vi "Drive Train Charts.vi"() -> ()   [LabVIEW 2016]
uses:
  <vilib>/Rock Robotics/Network Tables/NT Read Number.vi
panel:
  out "Right Target":dbl(graph)
  out "Right Throttle":dbl(graph)
  out "Right Velocity":dbl(graph)
  out "Right Current":dbl(graph)
  out "Left Target":dbl(graph)
  out "Left Throttle":dbl(graph)
  out "Left Velocity":dbl(graph)
  out "Left Current":dbl(graph)
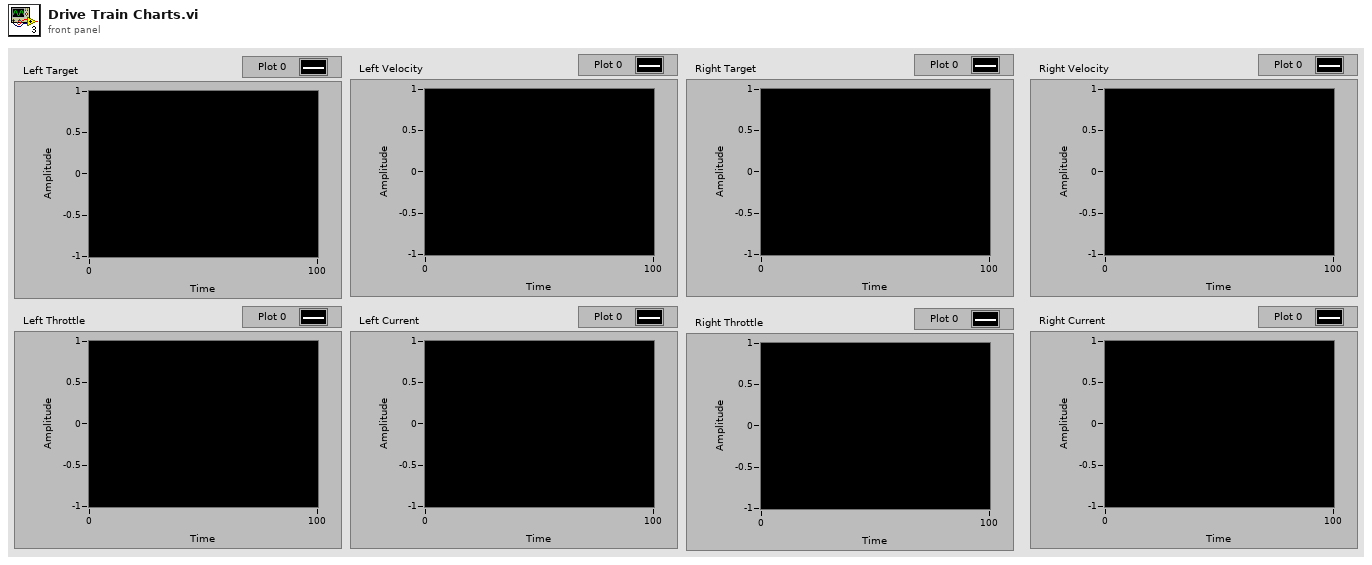
[diagram p1: front panel]
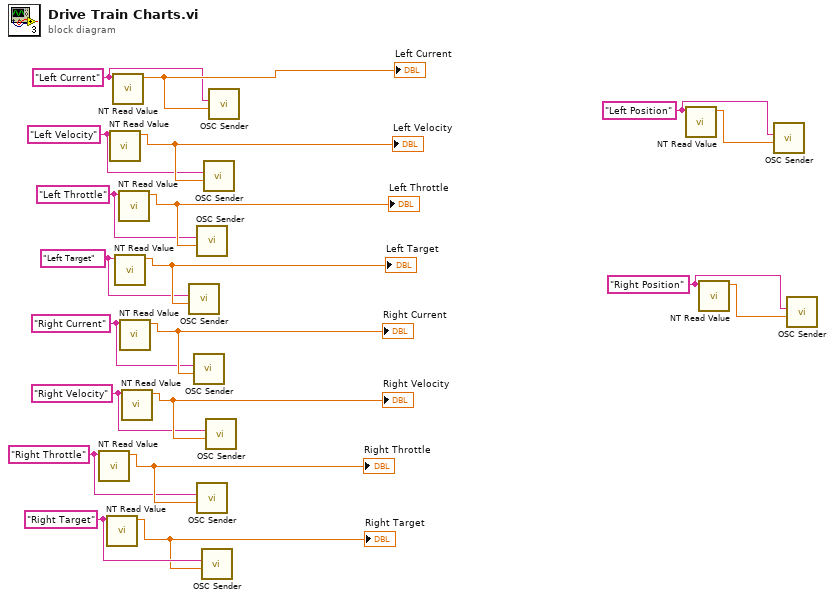
[diagram p0: block diagram]
diagram:
  w1 = "Right Position" ("Name")
  w3 = "Left Position" ("Name")
  w6 = "Right Target" ("Name")
  w7 = "Right Throttle" ("Name")
  w9 = "Right Velocity" ("Name")
  w11 = "Right Current" ("Name")
  w13 = "Left Target" ("Name")
  w15 = "Left Throttle" ("Name")
  w17 = "Left Velocity" ("Name")
  w19 = "Left Current" ("Name")
  n1 = call-poly <vilib>:"NT Read Value.vi"("Name"=w7) -> ("Numeric"=w8:dbl)  [unwired: 9 in, 1 out]
  "Right Throttle" <- w8
  n2 = call-poly <vilib>:"NT Read Value.vi"("Name"=w6) -> ("Numeric"=w5:dbl)  [unwired: 9 in, 1 out]
  "Right Target" <- w5
  n3 = call-poly <vilib>:"NT Read Value.vi"("Name"=w17) -> ("Numeric"=w18:dbl)  [unwired: 9 in, 1 out]
  "Left Velocity" <- w18
  n4 = call-poly <vilib>:"NT Read Value.vi"("Name"=w19) -> ("Numeric"=w20:dbl)  [unwired: 9 in, 1 out]
  "Left Current" <- w20
  n5 = call-poly <vilib>:"NT Read Value.vi"("Name"=w13) -> ("Numeric"=w14:dbl)  [unwired: 9 in, 1 out]
  "Left Target" <- w14
  n6 = call-poly <vilib>:"NT Read Value.vi"("Name"=w15) -> ("Numeric"=w16:dbl)  [unwired: 9 in, 1 out]
  "Left Throttle" <- w16
  n7 = call-poly <vilib>:"NT Read Value.vi"("Name"=w11) -> ("Numeric"=w12:dbl)  [unwired: 9 in, 1 out]
  "Right Current" <- w12
  n8 = call-poly <vilib>:"NT Read Value.vi"("Name"=w9) -> ("Numeric"=w10:dbl)  [unwired: 9 in, 1 out]
  "Right Velocity" <- w10
  n9 = call "OSC Sender.vi"("Value"=w14, "Label"=w13) -> ()  [unwired: 10 in]
  n10 = call "OSC Sender.vi"("Value"=w12, "Label"=w11) -> ()  [unwired: 10 in]
  n11 = call "OSC Sender.vi"("Value"=w16, "Label"=w15) -> ()  [unwired: 10 in]
  n12 = call "OSC Sender.vi"("Value"=w8, "Label"=w7) -> ()  [unwired: 10 in]
  n13 = call "OSC Sender.vi"("Value"=w5, "Label"=w6) -> ()  [unwired: 10 in]
  n14 = call "OSC Sender.vi"("Value"=w18, "Label"=w17) -> ()  [unwired: 10 in]
  n15 = call "OSC Sender.vi"("Value"=w10, "Label"=w9) -> ()  [unwired: 10 in]
  n16 = call "OSC Sender.vi"("Value"=w20, "Label"=w19) -> ()  [unwired: 10 in]
  n17 = call-poly <vilib>:"NT Read Value.vi"("Name"=w3) -> ("Numeric"=w4:dbl)  [unwired: 9 in, 1 out]
  n18 = call-poly <vilib>:"NT Read Value.vi"("Name"=w1) -> ("Numeric"=w2:dbl)  [unwired: 9 in, 1 out]
  n19 = call "OSC Sender.vi"("Value"=w4, "Label"=w3) -> ()  [unwired: 10 in]
  n20 = call "OSC Sender.vi"("Value"=w2, "Label"=w1) -> ()  [unwired: 10 in]
